vi "CreateToolbarObject.vi"(0 "reference in":refnum<class "SequenceDiagramGraph.lvclass">, 2 "GraphButton":u32, 5 "error in (no error)":errorcluster) -> (14 "reference out":refnum<class "SequenceDiagramGraph.lvclass">, 15 "toolType":T1, 16 "Edge":refnum<class "AbstractEdge.lvclass">, 17 "Node":refnum<class "AbstractNode.lvclass">, 18 "ButtonNameCompressed)":string, 19 "error out":errorcluster)   [LabVIEW 2020, in "SequenceDiagramGraph.lvclass"]
uses:
  <resource>/Framework/Providers/Open_GDS/UML/SequenceDiagramGraph_class/SequenceDiagramGraph.lvclass
  <resource>/Framework/Providers/Open_GDS/UML/UMLEditor/UMLEditor tooltype.ctl
  <resource>/Framework/Providers/Open_GDS/UML/AbstractEdge_class/AbstractEdge.lvclass
  <resource>/Framework/Providers/Open_GDS/UML/AbstractNode_class/AbstractNode.lvclass
  <resource>/Framework/Providers/Open_GDS/UML/ArrowHead_class/ArrowHeadType.ctl
  <resource>/Framework/Providers/Open_GDS/UML/BentStyle_class/BentStyleType.ctl
  <resource>/Framework/Providers/Open_GDS/UML/LineStyle_class/LineStyleType.ctl
  <resource>/Framework/Providers/Open_GDS/UML/Graph_class/ToolbarButtonType.ctl
  <resource>/Framework/Providers/Open_GDS/UML/ImplicitParameterNode_class/ImplicitParameterNode.lvclass
  C:/Program Files (x86)/National Instruments/LabVIEW 2020/resource/Framework/Providers/Open_GDS/UML/RectangularNode_class/RectangularNode.lvclass
  <resource>/Framework/Providers/Open_GDS/UML/CallNode_class/CallNode.lvclass
  <resource>/Framework/Providers/Open_GDS/UML/NoteNode_class/NoteNode.lvclass
  <resource>/Framework/Providers/Open_GDS/UML/CallEdge_class/CallEdge.lvclass
  C:/Program Files (x86)/National Instruments/LabVIEW 2020/resource/Framework/Providers/Open_GDS/UML/GeneralPathEdge_class/GeneralPathEdge.lvclass
  <resource>/Framework/Providers/Open_GDS/UML/NoteEdge_class/NoteEdge.lvclass
  <resource>/Framework/Providers/Open_GDS/UML/GeneralPathEdge_class/GeneralPathEdge.lvclass
  C:/Program Files (x86)/National Instruments/LabVIEW 2020/resource/Framework/Providers/Open_GDS/UML/AbstractEdge_class/AbstractEdge.lvclass
  <resource>/Framework/Providers/Open_GDS/UML/RectangularNode_class/RectangularNode.lvclass
  C:/Program Files (x86)/National Instruments/LabVIEW 2020/resource/Framework/Providers/Open_GDS/UML/AbstractNode_class/AbstractNode.lvclass
  <resource>/Framework/Providers/Open_GDS/UML/ArrowHead_class/ArrowHead.lvclass
  <resource>/Framework/Providers/Open_GDS/UML/BentStyle_class/BentStyle.lvclass
  <resource>/Framework/Providers/Open_GDS/UML/LineStyle_class/LineStyle.lvclass
  <resource>/Framework/Providers/Open_GDS/UML/Graph_class/Graph.lvclass
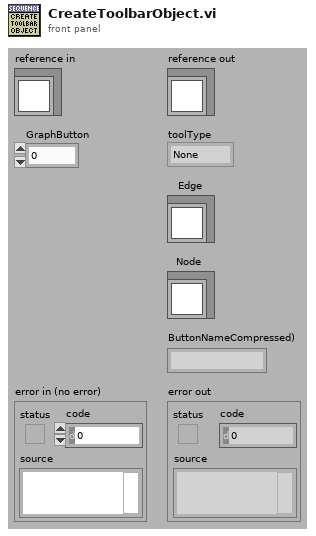
[diagram p1: front panel]
types:
  T1 = typedef "UMLEditor tooltype.ctl" = enum16{"None", "Node", "Edge"}
  T2 = typedef "Graph.lvclass/ToolbarButtonType.ctl" = cluster{"Text":string, "Type":T1}
  T3 = typedef "LineStyle.lvclass/LineStyleType.ctl" = enum16{"SOLID", "DOTTED"}
  T4 = typedef "BentStyle.lvclass/BentStyleType.ctl" = enum16{"STRAIGHT", "HV", "VH", "HVH", "VHV", "ARC"}
  T5 = typedef "ArrowHead.lvclass/ArrowHeadType.ctl" = enum16{"NONE", "TRIANGLE", "BLACK_TRIANGLE", "V", "HALF_V", "DIAMOND", "BLACK_DIAMOND"}
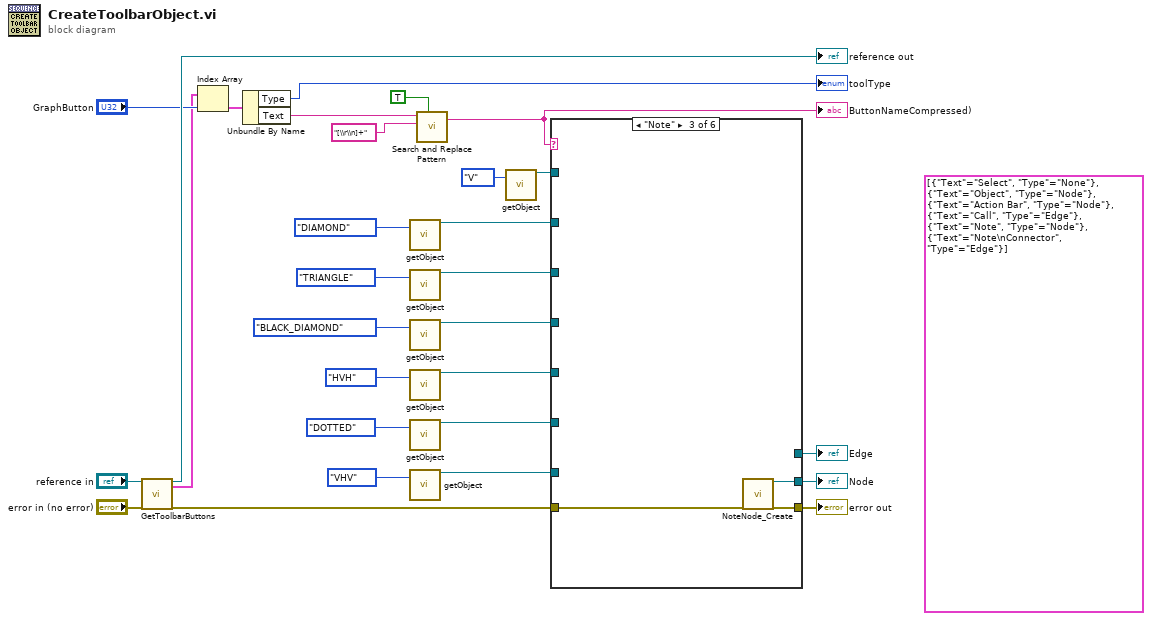
[diagram p0: block diagram]
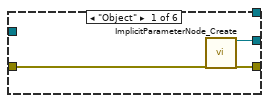
[diagram p2: hidden frame]
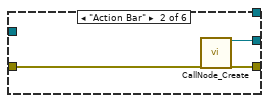
[diagram p3: hidden frame]
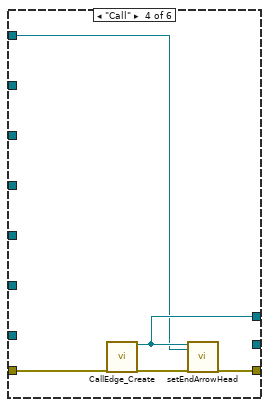
[diagram p4: hidden frame]
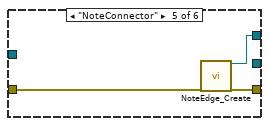
[diagram p5: hidden frame]
diagram:
  (unwired) T2[] [{"Text"="Select", "Type"=enum."None"}, {"Text"="Object", "Type"=enum."Node"}, {"Text"="Action Bar", "Type"=enum."Node"}, {"Text"="Call", "Type"=enum."Edge"}, {"Text"="Note", "Type"=enum."Node"}, {"Text"="Note\nConnector", "Type"=enum."Edge"}] ("ToolbarButtons")
  n1 = call-dynamic "GetToolbarButtons.vi"("reference in"="reference in", "error in (no error)"="error in (no error)") -> ("reference out"=→"reference out":refnum<class "SequenceDiagramGraph.lvclass">, "ToolbarButtons"=w20:T2[], "error out"=w11:errorcluster)  [unwired: 13 in, 2 out]
  n2 = Index Array(array=w20, index="GraphButton") -> (element=w19:T2)
  n3 = Unbundle By Name(w19) -> ("Type"=→"toolType":T1, "Text"=w3:string)
  n4 = call <resource>:"getObject.vi"("arrowHead"=ArrowHeadType."DIAMOND") -> ("reference out"=w5:refnum<class "ArrowHead.lvclass">)  [unwired: 1 in, 17 out]
  n5 = call <resource>:"getObject.vi"("arrowHead"=ArrowHeadType."TRIANGLE") -> ("reference out"=w7:refnum<class "ArrowHead.lvclass">)  [unwired: 1 in, 17 out]
  n6 = call <resource>:"getObject.vi"("arrowHead"=ArrowHeadType."BLACK_DIAMOND") -> ("reference out"=w4:refnum<class "ArrowHead.lvclass">)  [unwired: 1 in, 17 out]
  n7 = call <resource>:"getObject.vi"("bentStyle"=BentStyleType."HVH") -> ("reference out"=w6:refnum<class "BentStyle.lvclass">)  [unwired: 1 in, 17 out]
  n8 = call <resource>:"getObject.vi"("lineStyle"=LineStyleType."DOTTED") -> ("reference out"=w10:refnum<class "LineStyle.lvclass">)  [unwired: 1 in, 17 out]
  n9 = call <resource>:"getObject.vi"("bentStyle"=BentStyleType."VHV") -> ("reference out"=w8:refnum<class "BentStyle.lvclass">)  [unwired: 1 in, 17 out]
  n10 = call <vilib>:"Search and Replace Pattern.vi"("string"=w3, "regular expression (\"\")"="[\\r\\n]+" ("regular expression (\"\")"), "replace all? (F)"=TRUE) -> ("result string"=w21:string)  [unwired: 2 in, 1 out]
  "ButtonNameCompressed)" <- w21
  n11 = call <resource>:"getObject.vi"("arrowHead"=ArrowHeadType."V") -> ("reference out"=w9:refnum<class "ArrowHead.lvclass">)  [unwired: 1 in, 17 out]
  n12 = case shown="\"Note\"" w21 {
    tunnel: w11 -> [w32 w35 w38 w43 w46 w47]
    tunnel: [w31 w34 w37 w40 w45 w47] -> w28
    tunnel: [w30 w33 w36 _ _ _] -> w23
    tunnel: w10 -> [_ _ _ _ _ _]
    tunnel: w9 -> [_ _ _ w39 _ _]
    tunnel: w8 -> [_ _ _ _ _ _]
    tunnel: w7 -> [_ _ _ _ _ _]
    tunnel: w6 -> [_ _ _ _ _ _]
    tunnel: w5 -> [_ _ _ _ _ _]
    tunnel: w4 -> [_ _ _ _ _ _]
    tunnel: [_ _ _ w41 w44 _] -> w22
    frame "Object" {
      n13 = call <resource>:"ImplicitParameterNode_Create.vi"("error in (no error)"=w32) -> ("reference out"=w30:refnum<class "ImplicitParameterNode.lvclass">, "error out"=w31:errorcluster)  [unwired: 1 in, 16 out]
    }
    frame "Action Bar" {
      n14 = call <resource>:"CallNode_Create.vi"("error in (no error)"=w35) -> ("reference out"=w33:refnum<class "CallNode.lvclass">, "error out"=w34:errorcluster)  [unwired: 17 in]
    }
    frame "Note" {
      n15 = call <resource>:"NoteNode_Create.vi"("error in (no error)"=w38) -> ("reference out"=w36:refnum<class "NoteNode.lvclass">, "error out"=w37:errorcluster)  [unwired: 1 in, 16 out]
    }
    frame "Call" {
      n16 = call <resource>:"CallEdge_Create.vi"("error in (no error)"=w43) -> ("reference out"=w41:refnum<class "CallEdge.lvclass">, "error out"=w42:errorcluster)  [unwired: 1 in, 16 out]
      n17 = call-dynamic "setEndArrowHead.vi"("reference"=w41, "endArrowHead"=w39, "error in (no error)"=w42) -> ("error out"=w40:errorcluster)  [unwired: 15 in, 1 out]
    }
    frame "NoteConnector" {
      n18 = call <resource>:"NoteEdge_Create.vi"("error in (no error)"=w46) -> ("reference out"=w44:refnum<class "NoteEdge.lvclass">, "error out"=w45:errorcluster)  [unwired: 1 in, 16 out]
    }
    frame "Select", Default {
    }
  }
  "error out" <- w28
  "Edge" <- w22
  "Node" <- w23
